vi "Main.vi"() -> ()   [LabVIEW 2014]
uses:
  Elevator System/Elevator System.lvlib
panel:
  out "Elevator":T1(graph)
  out "Gripper":T2(graph)
  out "Gripper L":dbl(knob)
  out "Gripper R":dbl(knob) scale=0.0..100.0
  out "Elevator Right":dbl(slide) scale=0.0..100.0
  out "Elevator Left":dbl(slide) scale=0.0..100.0
  in  "RC Mode":bool
  in  "Cycle Mode":bool
  in  "Close":bool
  in  "Open":bool
  in  "Down":bool
  in  "Up":bool
  in  "Stop":bool
  in  "Score":bool
  in  "Pickup":bool
  in  "Home":bool
  in  "1":bool
  in  "2":bool
  in  "3":bool
  in  "4":bool
  in  "5":bool
  in  "6":bool
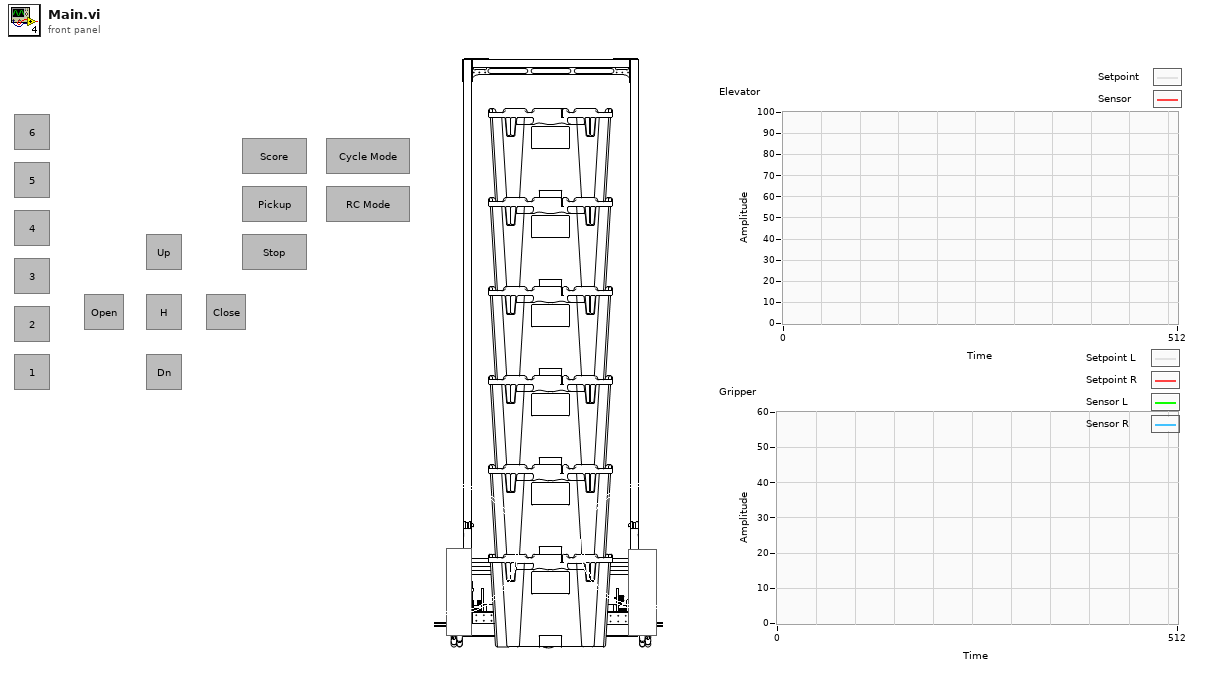
[diagram p1: front panel]
types:
  T1 = cluster{"Elevator SP":dbl, "Elevator Sensor":dbl}
  T2 = cluster{"Left":dbl, "Right":dbl, "Left":dbl, "Right":dbl}
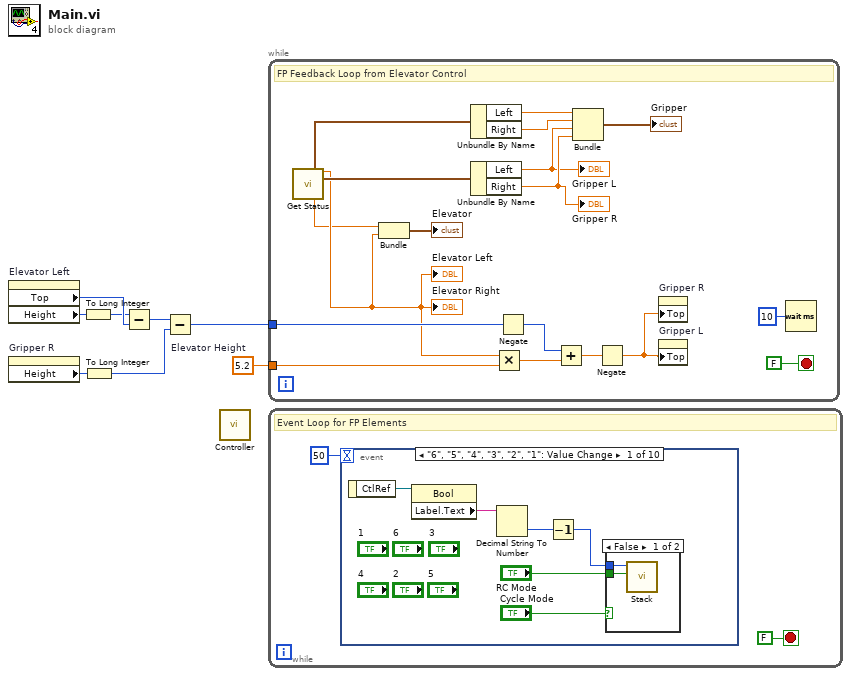
[diagram p0: block diagram]
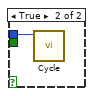
[diagram p2: hidden frame]
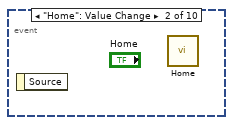
[diagram p3: hidden frame]
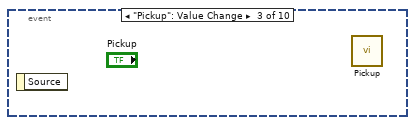
[diagram p4: hidden frame]
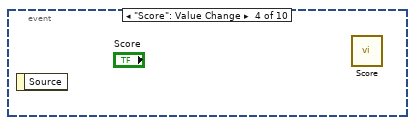
[diagram p5: hidden frame]
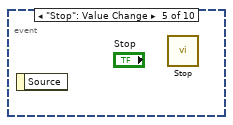
[diagram p6: hidden frame]
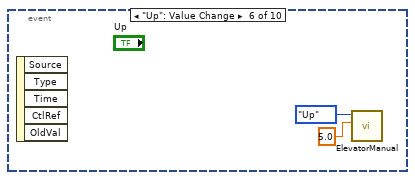
[diagram p7: hidden frame]
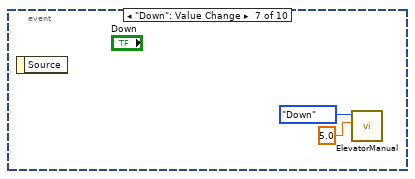
[diagram p8: hidden frame]
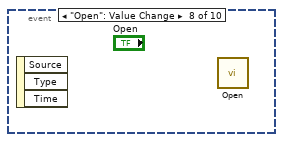
[diagram p9: hidden frame]
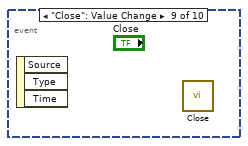
[diagram p10: hidden frame]
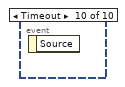
[diagram p11: hidden frame]
diagram:
  w8 = 5.2  # Elevator Height
  n1 = property on="Elevator Left" class="Slide (strict)"() -> ("Top"=w6:i32, "Height"=w7:u32)  [unwired: 2 in, 2 out]
  n2 = property on="Gripper R" class="Knob (strict)"() -> ("Height"=w4:u32)  [unwired: 2 in, 2 out]
  n3 = To Long Integer(number=w7) -> (32bit integer=w2:i32)
  n4 = To Long Integer(number=w4) -> (32bit integer=w1:i32)
  n5 = Subtract(x=w2, y=w6) -> (x-y=w5:i32)
  n6 = Subtract(x=w5, y=w1) -> (x-y=w3:i32)
  n7 = call "Controller.vi"() -> ()  [unwired: 12 in]
  n8 = while {
    tunnel: w3 -> [w20]
    tunnel: w8 -> [w19]
    stop <- FALSE stop-if-true
    # "FP Feedback Loop from Elevator Control"
    n9 = call "Get Status.vi"() -> ("Gripper SP"=w15:cluster{"Left":dbl, "Right":dbl}, "Elevator Sensor"=w11:dbl, "Gripper Sensor"=w18:cluster{"Left":dbl, "Right":dbl}, "Elevator SP"=w10:dbl)  [unwired: 9 in, 3 out]
    "Elevator Left" <- w11
    "Elevator Right" <- w11
    n10 = Bundle("Elevator SP"=w10, "Elevator Sensor"=w11) -> (→"Elevator":T1)  [unwired: 1 in]
    n11 = Unbundle By Name(w15) -> ("Left"=w14:dbl, "Right"=w13:dbl)
    n12 = Unbundle By Name(w18) -> ("Left"=w16:dbl, "Right"=w17:dbl)
    "Gripper R" <- w17
    "Gripper L" <- w16
    n13 = Multiply(x=w11, y=w19) -> (x*y=w22:dbl)
    n14 = Negate(x=w20) -> (-x=w23:i32)
    n15 = Add(x=w23, y=w22) -> (x+y=w21:dbl)
    n16 = Bundle("Left"=w14, "Right"=w13, "Left"=w16, "Right"=w17) -> (→"Gripper":T2)  [unwired: 1 in]
    n17 = Negate(x=w21) -> (-x=w24:dbl)
    n18 = property on="Gripper R" class="Knob (strict)"("Top"=w24) -> ()  [unwired: 2 in, 2 out]
    n19 = property on="Gripper L" class="Knob (strict)"("Top"=w24) -> ()  [unwired: 2 in, 2 out]
    n20 = Wait (ms)(milliseconds to wait=u32 10) -> ()  [unwired: 1 out]
  }
  n21 = while {
    stop <- FALSE stop-if-true
    # "Event Loop for FP Elements"
    n22 = event shown="[0] \"6\", \"5\", \"4\", \"3\", \"2\", \"1\": Value Change" {
      selector: _ -> [_ _ _ _ _ _ _ _ _ _]
      dyn-events: _ -> [_ _ _ _ _ _ _ _ _ _]
      timeout: 50 -> [_ _ _ _ _ _ _ _ _ _]
      event "6", "5", "4", "3", "2", "1": Value Change {
        n23 = event-data() -> ("CtlRef"=w34:refnum<vi>)  [unwired: 1 in]
        n24 = property class="Bool"(reference=w34) -> ("Label.Text"=w33:string)  [unwired: 1 in, 2 out]
        n25 = Decimal String To Number(string=w33) -> (number=w32:i32)  [unwired: 2 in, 1 out]
        n26 = Decrement(x=w32) -> (x-1=w31:i32)
        n27 = case shown="False" "Cycle Mode" {
          tunnel: w31 -> [w36 w37]
          tunnel: "RC Mode" -> [w35 _]
          frame False {
            n28 = call "Stack.vi"("RC?"=w35, "Teir"=w36) -> ()  [unwired: 10 in]
          }
          frame True {
            n29 = call "Cycle.vi"("Teir"=w37) -> ()  [unwired: 11 in]
          }
        }
      }
      event "Home": Value Change {
        n30 = event-data() -> ()  [unwired: 1 in, 1 out]
        n31 = call "Home.vi"() -> ()  [unwired: 12 in]
      }
      event "Pickup": Value Change {
        n32 = event-data() -> ()  [unwired: 1 in, 1 out]
        n33 = call "Pickup.vi"() -> ()  [unwired: 12 in]
      }
      event "Score": Value Change {
        n34 = event-data() -> ()  [unwired: 1 in, 1 out]
        n35 = call "Score.vi"() -> ()  [unwired: 12 in]
      }
      event "Stop": Value Change {
        n36 = event-data() -> ()  [unwired: 1 in, 1 out]
        n37 = call "Stop.vi"() -> ()  [unwired: 12 in]
      }
      event "Up": Value Change {
        n38 = event-data() -> ()  [unwired: 1 in, 5 out]
        n39 = call "ElevatorManual.vi"("Amount"=5.0, "Enum"=enum16{"Up", "Down"}."Up") -> ()  [unwired: 10 in]
      }
      event "Down": Value Change {
        n40 = event-data() -> ()  [unwired: 1 in, 1 out]
        n41 = call "ElevatorManual.vi"("Amount"=5.0, "Enum"=enum16{"Up", "Down"}."Down") -> ()  [unwired: 10 in]
      }
      event "Open": Value Change {
        n42 = event-data() -> ()  [unwired: 1 in, 3 out]
        n43 = call "Open.vi"() -> ()  [unwired: 12 in]
      }
      event "Close": Value Change {
        n44 = event-data() -> ()  [unwired: 1 in, 3 out]
        n45 = call "Close.vi"() -> ()  [unwired: 12 in]
      }
      event Timeout {
        n46 = event-data() -> ()  [unwired: 1 in, 1 out]
      }
    }
  }
